vi "InitHardware.vi"(8 "error in (no error)":errorcluster, 11 "XPS-RLD.lvclass":refnum<class "XPS-RLD.lvclass">) -> (0 "error out":errorcluster, 3 "XPS-RLD.lvclass":refnum<class "XPS-RLD.lvclass">)   [LabVIEW 2020, in "XPS-RLD.lvclass"]
uses:
  XPS-RLD/XPS-RLD.lvclass
  C:/GEECS/Developers Version/source/Device Drivers/NewportXPS/NewportXPS.lvclass
  XPS-RLD/XPS-RLD.lvclass/XPS-RLD.ctl
  ReadSettings.vi
  C:/Users/loasis.BELLANET/Downloads/XPS-UNIFIED/LabVIEW VIs/LabVIEW Source Code/Dll/Newport.XPS.CommandInterface.dll
  Users/loasis.BELLANET/Downloads/XPS-UNIFIED/LabVIEW VIs/LabVIEW Source Code/Dll/Newport.XPS.CommandInterface.dll
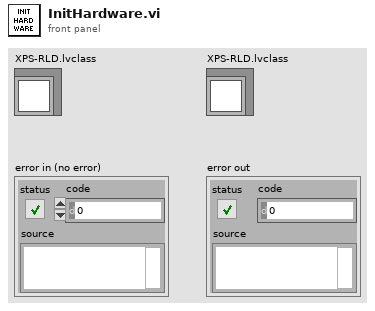
[diagram p1: front panel]
types:
  T1 = typedef "NewportXPS.lvclass/SettingsTypdef.ctl" = cluster{"ipaddress":string, "Position":cluster{"Axis 1":cluster{"Value":dbl, "Min":dbl, "Max":dbl, "StepSize":dbl, "Tolerance":dbl, "ValueActual":dbl}, "Axis 2":cluster{"Value":dbl, "Min":dbl, "Max":dbl, "StepSize":dbl, "Tolerance":dbl, "ValueActual":dbl}, "Axis 3":cluster{"Value":dbl, "Min":dbl, "Max":dbl, "StepSize":dbl, "Tolerance":dbl, "ValueActual":dbl}, "Axis 4":cluster{"Value":dbl, "Min":dbl, "Max":dbl, "StepSize":dbl, "Tolerance":dbl, "ValueActual":dbl}, "Axis 5":cluster{"Value":dbl, "Min":dbl, "Max":dbl, "StepSize":dbl, "Tolerance":dbl, "ValueActual":dbl}, "Axis 6":cluster{"Value":dbl, "Min":dbl, "Max":dbl, "StepSize":dbl, "Tolerance":dbl, "ValueActual":dbl}}, "PositionerName":cluster{"Axis 1":string, "Axis 2":string, "Axis 3":string, "Axis 4":string, "Axis 5":string, "Axis 6":string}, "FirstMoveSubtract":cluster{"Axis 1":cluster{"Value":dbl, "Min":dbl, "Max":dbl, "StepSize":dbl, "Tolerance":dbl, "ValueActual":dbl}, "Axis 2":cluster{"Value":dbl, "Min":dbl, "Max":dbl, "StepSize":dbl, "Tolerance":dbl, "ValueActual":dbl}, "Axis 3":cluster{"Value":dbl, "Min":dbl, "Max":dbl, "StepSize":dbl, "Tolerance":dbl, "ValueActual":dbl}, "Axis 4":cluster{"Value":dbl, "Min":dbl, "Max":dbl, "StepSize":dbl, "Tolerance":dbl, "ValueActual":dbl}, "Axis 5":cluster{"Value":dbl, "Min":dbl, "Max":dbl, "StepSize":dbl, "Tolerance":dbl, "ValueActual":dbl}, "Axis 6":cluster{"Value":dbl, "Min":dbl, "Max":dbl, "StepSize":dbl, "Tolerance":dbl, "ValueActual":dbl}}}
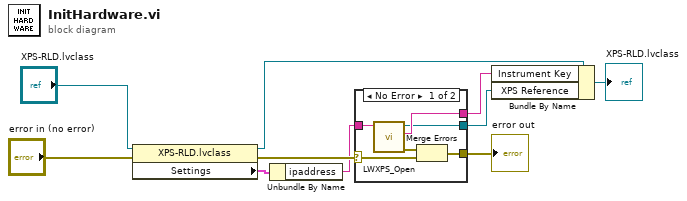
[diagram p0: block diagram]
diagram:
  n1 = property class="XPS-RLD.lvclass"(reference="XPS-RLD.lvclass", error in="error in (no error)") -> (reference out=w2:refnum<class "XPS-RLD.lvclass">, error out=w7:errorcluster, "Settings"=w6:T1)
  n2 = Unbundle By Name(w6) -> ("ipaddress"=w5:string)
  n3 = case shown="No Error" w7 {
    selector: w7 -> [w12 w17]
    tunnel: w5 -> [w16 _]
    tunnel: [w15 _] -> w4
    tunnel: [w14 _] -> w1
    tunnel: [w11 w17] -> w3
    frame No Error {
      n4 = call "LWXPS_Open.vi"("Instrument Key IN"=w16) -> ("LabVIEW error OUT"=w13:errorcluster, "Instrument Key OUT"=w15:string, "XPS Reference OUT"=w14:refnum<k24>)  [unwired: 3 in, 1 out]
      n5 = Merge Errors(w13, w12) -> (w11:errorcluster)
    }
    frame Error {
    }
  }
  "error out" <- w3
  n6 = Bundle By Name(cluster=w2, "Instrument Key"=w4, "XPS Reference"=w1) -> (→"XPS-RLD.lvclass":refnum<class "XPS-RLD.lvclass">)
